vi "MGI Write Spreadsheet File.vi"(4 "Dialog pattern (*.txt)":string="*.txt", 5 "Data Format (%#_8g)":string="%#_8g", 6 "Existing File Behavior":T1, 7 "Delimiter (Tab)":string="\t", 8 "Error In":errorcluster, 9 "Data[row][col]":dbl[][](array[numeric]), 10 "Header Lines[row][col]":string[][](array[string]), 11 "Path":path) -> (0 "Error Out":errorcluster, 1 "File Pos Out":i64, 2 "Created?":bool, 3 "Duplicate Path":path)   [LabVIEW 2020]
doc: "Creates or opens the specified spreadsheet file and writes the specified data to the end of the file. This VI is similar to the vi.lib\\Write Spreadsheet File.vi, but it includes headers.\nBy default, headers are only written if the file is created new. Wire true to \"Append Headers to existing files?\" to add them to existing files as well.\n\nAuthored by Shawn Walpole\nsupport@mooregoodideas.com\nwww.mooregoodideas.com\n\nCopyright (c) 2010, Moore Good Ideas, Inc.\n\nAll rights reserved.\n\nRedistribution and use in source and binary forms, with or without modification, are permitted provided that the following conditions are met:\n\n * Redistributions of source code must retain the above copyright notice, this list of conditions and the following disclaimer.\n * Redistributions in binary form must reproduce the above copyright notice, this list of conditions and the following disclaimer in the documentation and/or other materials provided with the distribution.\n * Neither the name of Moore Good Ideas, Inc. nor the names of its contributors may be used to endorse or promote products derived from this software without specific prior written permission.\n\nTHIS SOFTWARE IS PROVIDED BY THE COPYRIGHT HOLDERS AND CONTRIBUTORS \"AS IS\" AND ANY EXPRESS OR IMPLIED WARRANTIES, INCLUDING, BUT NOT LIMITED TO, THE IMPLIED WARRANTIES OF MERCHANTABILITY AND FITNESS FOR A PARTICULAR PURPOSE ARE DISCLAIMED. IN NO EVENT SHALL THE COPYRIGHT OWNER OR CONTRIBUTORS BE LIABLE FOR ANY DIRECT, INDIRECT, INCIDENTAL, SPECIAL, EXEMPLARY, OR CONSEQUENTIAL DAMAGES (INCLUDING, BUT NOT LIMITED TO, PROCUREMENT OF SUBSTITUTE GOODS OR SERVICES; LOSS OF USE, DATA, OR PROFITS; OR BUSINESS INTERRUPTION) HOWEVER CAUSED AND ON ANY THEORY OF LIABILITY, WHETHER IN CONTRACT, STRICT LIABILITY, OR TORT (INCLUDING NEGLIGENCE OR OTHERWISE) ARISING IN ANY WAY OUT OF THE USE OF THIS SOFTWARE, EVEN IF ADVISED OF THE POSSIBILITY OF SUCH DAMAGE."
uses:
  MGI Write Spreadsheet Behavior Enum.ctl
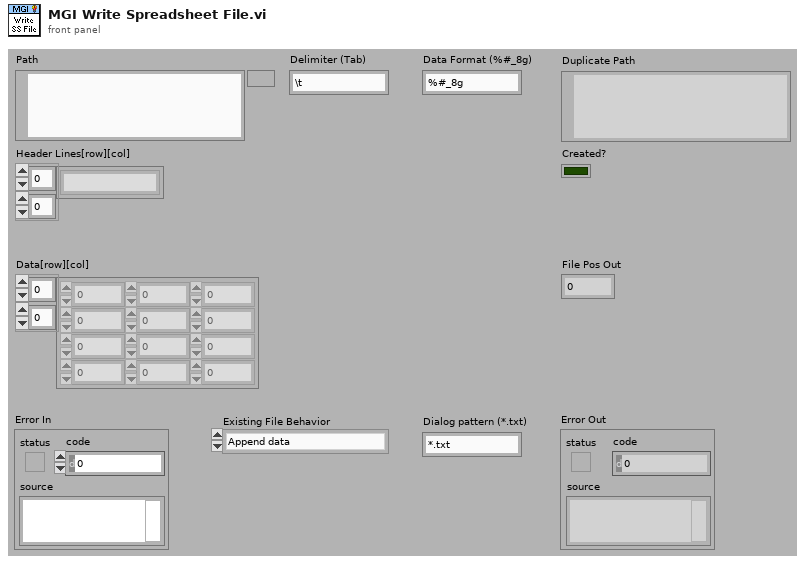
[diagram p1: front panel]
types:
  T1 = typedef "MGI Write Spreadsheet Behavior Enum.ctl" = enum16{"Append data", "Append headers and data", "Overwrite"}
  T2 = enum16{"open", "replace", "create", "open or create", "replace or create", "replace or create with confirmation"}
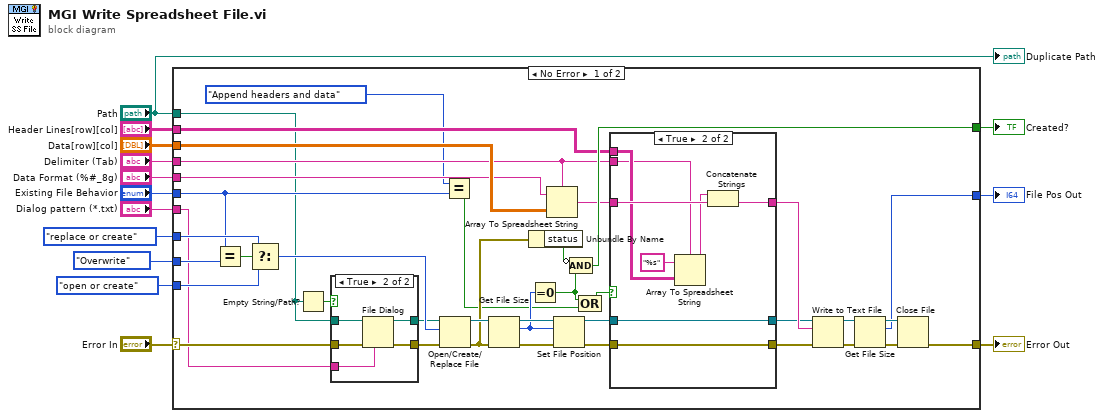
[diagram p0: block diagram]
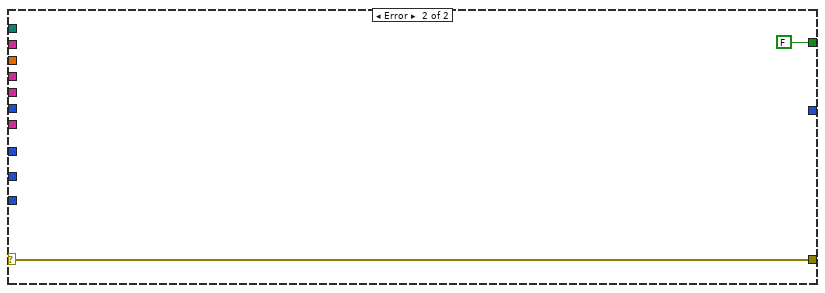
[diagram p4: hidden frame]
diagram:
  n1 = case shown="No Error" "Error In" {
    selector: "Error In" -> [w25 w73]
    tunnel: [w41 w73] -> w13
    tunnel: "Path" -> [w22 _]
    tunnel: "Header Lines[row][col]" -> [w40 _]
    tunnel: [w50 FALSE] -> w11
    tunnel: "Delimiter (Tab)" -> [w39 _]
    tunnel: "Data Format (%#_8g)" -> [w46 _]
    tunnel: "Data[row][col]" -> [w47 _]
    tunnel: "Existing File Behavior" -> [w29 _]
    tunnel: "Dialog pattern (*.txt)" -> [w20 _]
    tunnel: T2."open or create" ("operation (0:open)") -> [w34 _]
    tunnel: T2."replace or create" ("operation (0:open)") -> [w33 _]
    tunnel: MGI_Write_Spreadsheet_Behavior_Enum."Overwrite" ("y") -> [w28 _]
    tunnel: [w15 _] -> w1
    frame No Error {
      n2 = Equal?(x=w29, y=w28) -> (x = y?=w35:bool)
      n3 = Select(t=w33, s=w35, f=w34) -> (s? t:f=w32:T2)
      n4 = Empty String/Path?(string/path=w22) -> (empty?=w23:bool)
      n5 = case shown="True" w23 {
        tunnel: w25 -> [w55 w60]
        tunnel: [w55 w59] -> w24
        tunnel: w22 -> [w54 w58]
        tunnel: [w54 w56] -> w21
        tunnel: w20 -> [_ w57]
        frame False {
        }
        frame True {
          n6 = File Dialog(6:w57, 8:w60, 11:w58) -> (0:w59:errorcluster, 3:w56:path)  [unwired: 4 in, 2 out]
        }
      }
      n7 = Open/Create/Replace File(file path (use dialog)=w21, error in=w24, operation (0:open)=w32) -> (refnum out=w31:refnum<file>, error out=w30:errorcluster)  [unwired: 3 in, 1 out]
      n8 = Equal?(x=MGI_Write_Spreadsheet_Behavior_Enum."Append headers and data" ("y"), y=w29) -> (x = y?=w26:bool)
      n9 = Get File Size(file=w31, error in=w30) -> (refnum out=w53:refnum<file>, size (in bytes)=w36:i64, 0:w52:errorcluster)
      n10 = Unbundle By Name(w30) -> ("status"=w51:bool)
      n11 = Equal To 0?(x=w36) -> (x = 0?=w38:bool)
      n12 = Array To Spreadsheet String(delimiter (Tab)=w39, array=w47, 3:w46) -> (spreadsheet string=w45:string)
      n13 = Set File Position(offset (in bytes) (0)=w36, refnum=w53, error in=w52) -> (refnum out=w48:refnum<file>, error out=w49:errorcluster)  [unwired: 1 in]
      n14 = Compound Arithmetic op=AND(invert w51, w38) -> (w50:bool)
      n15 = Compound Arithmetic op=OR(w38, w26) -> (w37:bool)
      n16 = case shown="True" w37 {
        tunnel: w49 -> [w61 w68]
        tunnel: w48 -> [w62 w67]
        tunnel: w45 -> [w63 w70]
        tunnel: [w63 w69] -> w44
        tunnel: [w62 w67] -> w43
        tunnel: [w61 w68] -> w42
        tunnel: w40 -> [_ w66]
        tunnel: w39 -> [_ w65]
        frame False {
        }
        frame True {
          n17 = Array To Spreadsheet String(delimiter (Tab)=w65, array=w66, 3:"%s" ("format string")) -> (spreadsheet string=w64:string)
          n18 = Concatenate Strings(w64, w70) -> (w69:string)
        }
      }
      n19 = Write to Text File(file (use dialog)=w43, text=w44, error in=w42) -> (refnum out=w19:refnum<file>, error out=w18:errorcluster)  [unwired: 1 in, 1 out]
      n20 = Get File Size(file=w19, error in=w18) -> (refnum out=w16:refnum<file>, size (in bytes)=w15:i64, 0:w17:errorcluster)
      n21 = Close File(refnum=w16, error in=w17) -> (error out=w41:errorcluster)  [unwired: 1 out]
    }
    frame Error {
    }
  }
  "Error Out" <- w13
  "Created?" <- w11
  "File Pos Out" <- w1
  "Duplicate Path" <- "Path"
